vi "Test Create Instrument.vi"() -> ()   [LabVIEW 2016]
uses:
  Example Instrument.lvclass
  C:/user/patrick/hg/levylab_inst del/lvsrc/SMOs/Instrument/Instrument.lvclass
  Instrument/Instrument.lvclass
  C:/Program Files (x86)/National Instruments/LabVIEW 2016/vi.lib/JKI/JKI SMO/SMO/SMO.lvclass
  <vilib>/JKI/JKI SMO/SMO/SMO.lvclass
panel:
  in  "Example?\nT = Instrumnt.Example Instrument\nF = Instrument.lvclass":bool
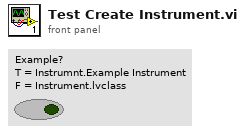
[diagram p1: front panel]
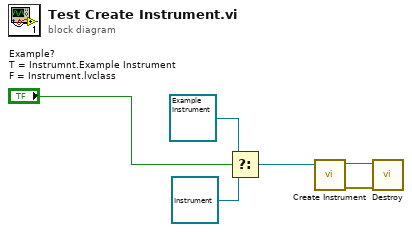
[diagram p0: block diagram]
diagram:
  n1 = Select(t=refnum<class "Example Instrument.lvclass"> refnum ("Example Instrument.lvclass"), s="Example?\nT = Instrumnt.Example Instrument\nF = Instrument.lvclass", f=refnum<class "Instrument.lvclass"> refnum ("Instrument.lvclass")) -> (s? t:f=w4:refnum<class "Instrument.lvclass">)
  n2 = call-dynamic "Create Instrument.vi"("Instrument in"=w4) -> ("error out"=w3:errorcluster, "Instrument out"=w2:refnum<class "Instrument.lvclass">)  [unwired: 9 in]
  n3 = call <vilib>:"Destroy.vi"("error in (no error)"=w3, "SMO"=w2) -> ()  [unwired: 9 in, 1 out]
